vi "RotateVector_.vi"(2 "Angle":dbl, 3 "X":dbl, 4 "Y":dbl) -> (0 "X'":dbl, 1 "Y'":dbl)   [LabVIEW 2015]
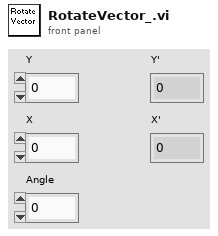
[diagram p1: front panel]
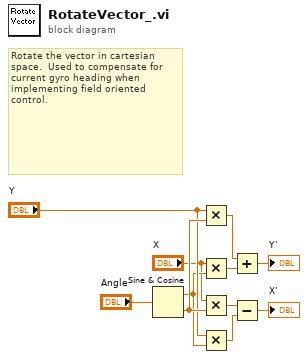
[diagram p0: block diagram]
diagram:
  # "Rotate the vector in cartesian space.  Used to compensate for current gyro heading when implementing field oriented control."
  n1 = Sine & Cosine(0:"Angle") -> (1:w6:dbl, 2:w8:dbl)
  n2 = Multiply(x="Y", y=w8) -> (x*y=w9:dbl)
  n3 = Multiply(x="X", y=w6) -> (x*y=w10:dbl)
  n4 = Multiply(x="X", y=w8) -> (x*y=w2:dbl)
  n5 = Multiply(x="Y", y=w6) -> (x*y=w3:dbl)
  n6 = Add(x=w9, y=w10) -> (x+y=→"Y'":dbl)
  n7 = Subtract(x=w2, y=w3) -> (x-y=→"X'":dbl)
